vi "Copy.vi"(8 "error in (no error)":errorcluster, 9 "size":u64 format="%d bytes", 10 "dst Pointer in":refnum<class "Pointer.lvclass">, 11 "src Pointer in":refnum<class "Pointer.lvclass">) -> (0 "error out":errorcluster, 1 "size":u64 format="%d bytes", 2 "dst Pointer out":refnum<class "Pointer.lvclass">, 3 "src Pointer out":refnum<class "Pointer.lvclass">)   [LabVIEW 2020, in "Memory Manager.lvlib" / "Pointer.lvclass"]
doc: "Copies <b>size</b> bytes from <b>src Pointer</b> to <b>dst Pointer</b>."
uses:
  Pointer.lvclass
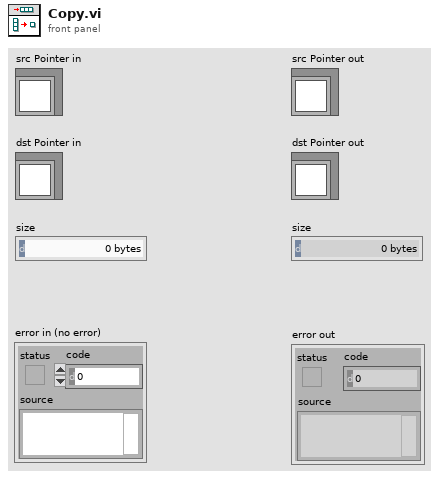
[diagram p1: front panel]
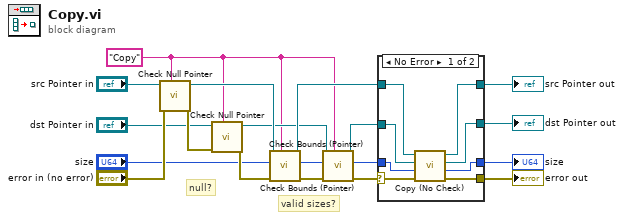
[diagram p0: block diagram]
diagram:
  w4 = "Copy" ("source vi name")
  # "valid sizes?"
  # "null?"
  n1 = call "Check Null Pointer.vi"("source vi name"=w4, "error in (no error)"="error in (no error)", "Pointer in"="src Pointer in") -> ("error out"=w8:errorcluster, "Pointer out"=w10:refnum<class "Pointer.lvclass">)  [unwired: 7 in]
  n2 = call "Check Null Pointer.vi"("source vi name"=w4, "error in (no error)"=w8, "Pointer in"="dst Pointer in") -> ("error out"=w6:errorcluster, "Pointer out"=w9:refnum<class "Pointer.lvclass">)  [unwired: 7 in]
  n3 = call "Check Bounds (Pointer).vi"("source vi name"=w4, "error in (no error)"=w6, "size"="size", "Pointer in"=w10) -> ("error out"=w15:errorcluster, "size"=w3:u64, "Pointer out"=w13:refnum<class "Pointer.lvclass">)  [unwired: 4 in, 1 out]
  n4 = call "Check Bounds (Pointer).vi"("source vi name"=w4, "error in (no error)"=w15, "size"=w3, "Pointer in"=w9) -> ("error out"=w14:errorcluster, "size"=w2:u64, "Pointer out"=w12:refnum<class "Pointer.lvclass">)  [unwired: 4 in, 1 out]
  n5 = case shown="No Error" w14 {
    selector: w14 -> [w20 w28]
    tunnel: [w24 w29] -> w19
    tunnel: w2 -> [w25 w29]
    tunnel: w13 -> [w27 w31]
    tunnel: w12 -> [w26 w30]
    tunnel: [w22 w31] -> w18
    tunnel: [w21 w30] -> w17
    tunnel: [w23 w28] -> w16
    frame No Error {
      n6 = call "Copy (No Check).vi"("error in (no error)"=w20, "bytes to copy"=w25, "dst Pointer in"=w26, "src Pointer in"=w27) -> ("error out"=w23:errorcluster, "bytes to copy"=w24:u64, "dst Pointer out"=w21:refnum<class "Pointer.lvclass">, "src Pointer out"=w22:refnum<class "Pointer.lvclass">)  [unwired: 4 in]
    }
    frame Error {
    }
  }
  "error out" <- w16
  "src Pointer out" <- w18
  "dst Pointer out" <- w17
  "size" <- w19
